vi "EXA shm issue Command disable LV.vi"(8 "error in (no error)":errorcluster, 11 "command_disable_Ctl":cluster{"state":u8}) -> (0 "error out":errorcluster, 2 "function return":i32, 3 "command_disable_Ctl out":cluster{"state":u8})   [LabVIEW 2016, in "SALLV_EXA.lvlib"]
doc: "int EXA_shm_issueCommand_disableLV(EXA_command_disableLV *command_disable_Ctl );"
uses:
  SALLV_EXA.lvlib
  SALLV_EXA.so
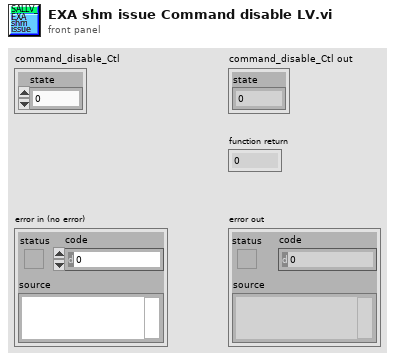
[diagram p1: front panel]
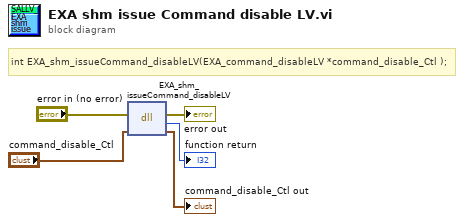
[diagram p0: block diagram]
diagram:
  # "int EXA_shm_issueCommand_disableLV(EXA_command_disableLV *command_disable_Ctl );"
  n1 = dll-call lib="home/plotz/SALLV_EXA/SALLV_EXA.*" fn="EXA_shm_issueCommand_disableLV"(error in="error in (no error)", "command_disable_Ctl"="command_disable_Ctl") -> (error out=→"error out":errorcluster, →"function return":i32, "command_disable_Ctl"=→"command_disable_Ctl out":cluster{"state":u8})  [unwired: 2 in, 1 out]
